vi "3.chaine de caractère_GJE.vi"() -> ()   [LabVIEW 2018]
panel:
  out "Prénom":string
  out "Résidue":bool
  out "Nom":string
  in  "Nom brut":string
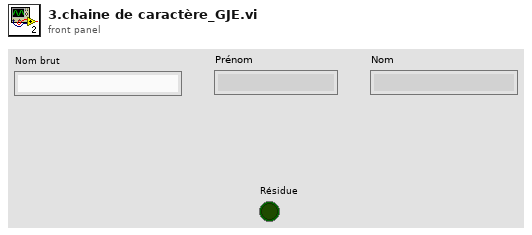
[diagram p1: front panel]
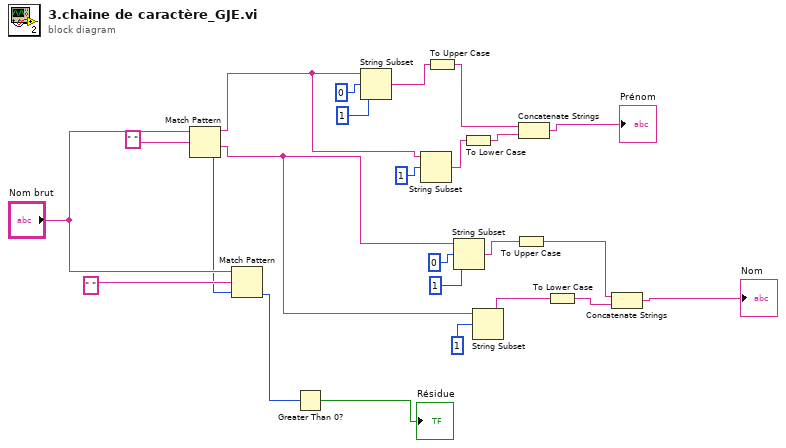
[diagram p0: block diagram]
diagram:
  n1 = Match Pattern(string="Nom brut", regular expression=" " ("string")) -> (before substring=w1:string, after substring=w13:string, offset past match=w17:i32)  [unwired: 1 in, 1 out]
  n2 = Match Pattern(string="Nom brut", regular expression=" " ("string"), offset (0)=w17) -> (offset past match=w16:i32)  [unwired: 3 out]
  n3 = Greater Than 0?(x=w16) -> (x > 0?=→"Résidue":bool)
  n4 = String Subset(string=w1, offset (0)=0, length (rest)=1 ("length (rest)")) -> (substring=w11:string)
  n5 = String Subset(string=w1, offset (0)=1) -> (substring=w12:string)  [unwired: 1 in]
  n6 = To Upper Case(1:w11) -> (0:w10:string)
  n7 = String Subset(string=w13, offset (0)=0, length (rest)=1 ("length (rest)")) -> (substring=w8:string)
  n8 = To Lower Case(string=w12) -> (all lower case string=w9:string)
  n9 = String Subset(string=w13, offset (0)=1) -> (substring=w5:string)  [unwired: 1 in]
  n10 = To Upper Case(1:w8) -> (0:w7:string)
  n11 = Concatenate Strings(w10, w9) -> (→"Prénom":string)
  n12 = To Lower Case(string=w5) -> (all lower case string=w6:string)
  n13 = Concatenate Strings(w7, w6) -> (→"Nom":string)
